vi "NoisySine.vi"() -> ()   [LabVIEW 2014]
uses:
  <vilib>/imath/engines/lvmath2/RunTimeEngine/Managers/WorkSpace/UID Generator.vi
  <vilib>/imath/engines/lvmath2/RunTimeEngine/RangeToken/NIMS_Range.vi
  <instcachedir>/0/NIMS_Range_9BCE657718DF4976A877346C61F22738.lvgen/NIMS_Range_9BCE657718DF4976A877346C61F22738_000.vi
  <vilib>/imath/engines/lvmath2/RunTimeEngine/RunTimeType/NIMS_RunTimeType_From StrictType (excl LVString).vi
  <instcachedir>/0/NIMS_RunTimeType_From StrictType (excl LVString)_15A5391EEA9C4AACB9955AC755B83D29.lvgen/NIMS_RunTimeType_From StrictType (excl LVString)_15A5391EEA9C4AACB9955AC755B83D29_000.vi
  <vilib>/imathl/engines/lvmath/Functions/Error Handling/Create Error.vi
  <vilib>/imath/engines/lvmath2/RunTimeEngine/LocalVariableDefStatement/MC_LocalVariableDefStatement_Display.vi
  <vilib>/imath/engines/lvmath2/RunTimeEngine/BuiltInFunctions/randnormal/NIMS_randnormal(1,I32).vi
  <vilib>/imath/engines/lvmath2/RunTimeEngine/ArithmeticOperatorToken/NIMS_ArithmeticOperator_plus.vi
  <instcachedir>/0/NIMS_ArithmeticOperator_plus_48D6EAACA5D645B09F7EC9C016C2DEA8.lvgen/NIMS_ArithmeticOperator_plus_48D6EAACA5D645B09F7EC9C016C2DEA8_004.vi
  <vilib>/imath/engines/lvmath2/RunTimeEngine/ErrorHandling/NIMS_Error From Error Code.vi
  <vilib>/imath/engines/lvmath2/RunTimeEngine/Managers/SymbolTable/Clear UID.vi
  <vilib>/imath/engines/lvmath2/RunTimeEngine/NodeEndStatement/NIMS_NodeEndStatement_Output.vi
  <instcachedir>/0/NIMS_NodeEndStatement_Output_53EC0D466D134D7ABD903AC30B43404B.lvgen/NIMS_NodeEndStatement_Output_53EC0D466D134D7ABD903AC30B43404B_005.vi
  <vilib>/imath/engines/lvmath2/RunTimeEngine/ErrorHandling/NIMS_Finalize Error.vi
  <vilib>/imath/engines/lvmath2/RunTimeEngine/Managers/SymbolTable/NIMS_WorkSpace.lvlib
panel:
  in  "Frequency":dbl format="%#_13g"
  in  "Number of Samples":i32
  out "XY Graph":cluster{dbl[], dbl[]}(graph)
  # "This generates an approximation of a real but noisy signal of specified frequency\nIncreased number of samples increases apparent resolution of the wave (reduces\nnoise effect)"
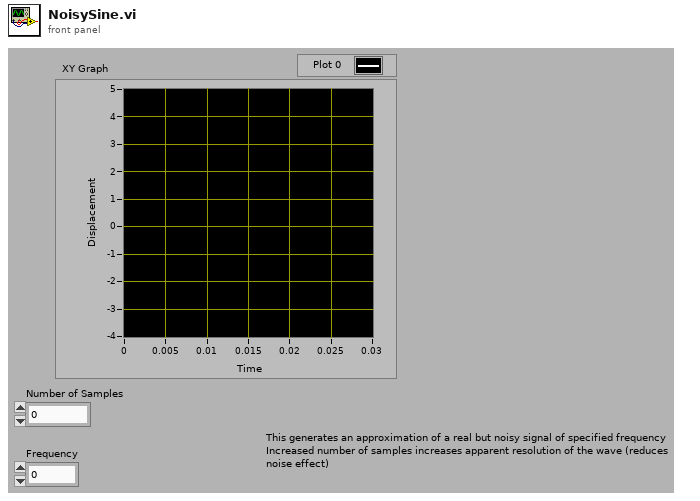
[diagram p1: front panel]
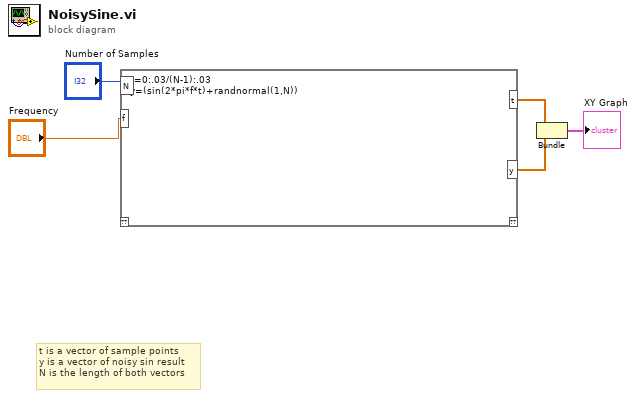
[diagram p0: block diagram]
diagram:
  # "t is a vector of sample points\ny is a vector of noisy sin result\nN is the length of both vectors"
  n1 = mathscript code="t=0:.03/(N-1):.03\ny=(sin(2*pi*f*t)+randnormal(1,N))"("N"="Number of Samples", "f"="Frequency") -> ("t"=w5:dbl[], "y"=w4:dbl[])  [unwired: 1 in, 1 out]
  n2 = Bundle("t"=w5, "y"=w4) -> (→"XY Graph":cluster{"t":dbl[], "y":dbl[]})  [unwired: 1 in]
